vi "Perform Action.vi"(7 "Action":T1, 8 "error in (no error)":errorcluster, 11 "Item in":refnum<class "Item.lvclass">) -> (0 "error out":errorcluster, 2 "Action Performed?":bool, 3 "Item out":refnum<class "Item.lvclass">)   [LabVIEW 2020, in "Code Cleanup.lvlib" / "Item.lvclass"]
uses:
  Item.lvclass
  Item.lvclass/Item.ctl
  Code Cleanup.lvlib
  CTLs/Cleanup Action.ctl
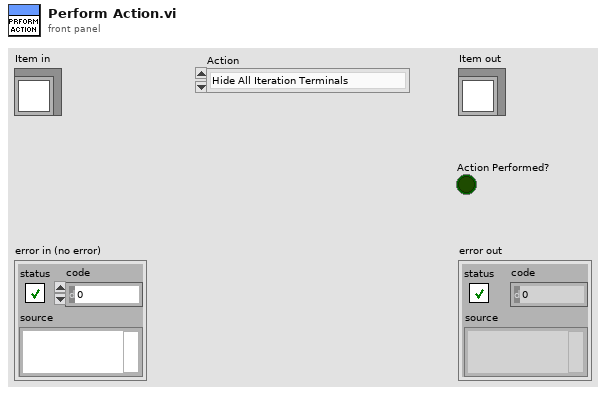
[diagram p1: front panel]
types:
  T1 = typedef "Code Cleanup.lvlib/Cleanup Action.ctl" = enum16{"Hide All Iteration Terminals", "Rename Window Title to VI Name", "Set Minimum Pane Size to (0,0)", "Set Origin to (0,0)", "Set Terminals to Required", "Fix VI Icon Properties", "Add Library Icon Layer", "Add VI Icon Layer", "Remove Icon Template", "Remove Autogrow from Structures", "Arrange Control Labels", "Format Control Labels", "Set Default FP BG Color", "Unshow Controls as Icons", "Set Modern Control Style", "Set Default Grid Sizes"}
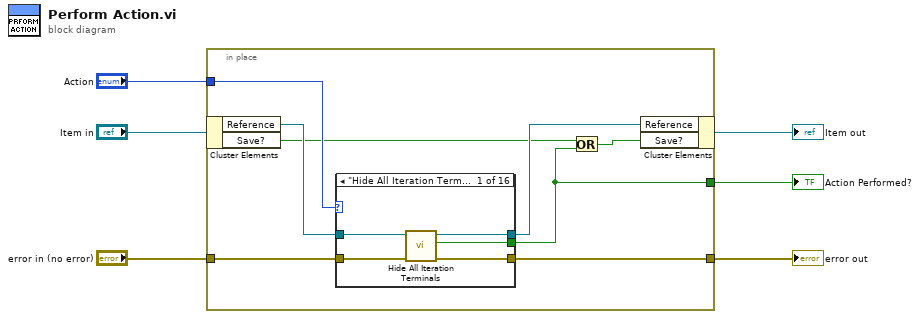
[diagram p0: block diagram]
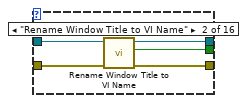
[diagram p2: hidden frame]
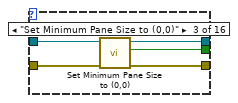
[diagram p3: hidden frame]
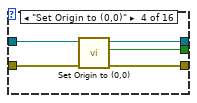
[diagram p4: hidden frame]
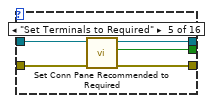
[diagram p5: hidden frame]
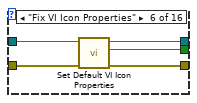
[diagram p6: hidden frame]
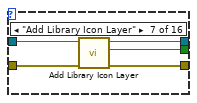
[diagram p7: hidden frame]
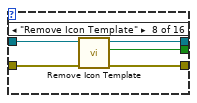
[diagram p8: hidden frame]
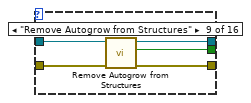
[diagram p9: hidden frame]
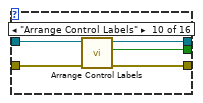
[diagram p10: hidden frame]
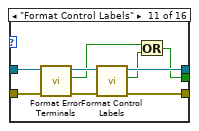
[diagram p11: hidden frame]
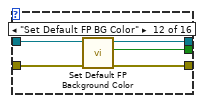
[diagram p12: hidden frame]
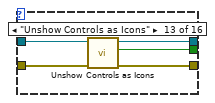
[diagram p13: hidden frame]
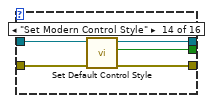
[diagram p14: hidden frame]
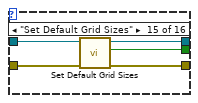
[diagram p15: hidden frame]
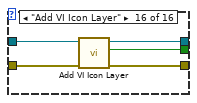
[diagram p16: hidden frame]
diagram:
  n1 = in-place {
    in-place-border: "Action" -> [w13]
    in-place-border: "error in (no error)" -> [w14]
    in-place-border: [w11] -> w2
    in-place-border: [w7] -> w1
    n2 = in-place-cluster #1("Item in") -> ("Reference"=w12:refnum<vi>, "Save?"=w9:bool)
    n3 = case shown="\"Hide All Iteration Terminals\"" w13 {
      tunnel: w14 -> [w19 w24 w29 w34 w39 w44 w49 w54 w59 w64 w72 w78 w83 w88 w93 w98]
      tunnel: w12 -> [w17 w22 w27 w32 w38 w42 w47 w52 w57 w62 w70 w76 w81 w86 w91 w96]
      tunnel: [w18 w23 w28 w33 w37 w43 w48 w53 w58 w63 w73 w77 w82 w87 w92 w97] -> w11
      tunnel: [w16 w21 w26 w31 w36 w41 w46 w51 w56 w61 w68 w75 w80 w85 w90 w95] -> w10
      tunnel: [w15 w20 w25 w30 w35 w40 w45 w50 w55 w60 w65 w74 w79 w84 w89 w94] -> w7
      frame "Hide All Iteration Terminals" {
        n4 = call "Hide All Iteration Terminals.vi"("error in (no error)"=w19, "VI Ref"=w17) -> ("error out"=w18:errorcluster, "Save?"=w15:bool, "VI Ref out"=w16:refnum<vi>)  [unwired: 7 in]
      }
      frame "Rename Window Title to VI Name" {
        n5 = call "Rename Window Title to VI Name.vi"("error in (no error)"=w24, "VI Ref"=w22) -> ("error out"=w23:errorcluster, "Save?"=w20:bool, "VI Ref out"=w21:refnum<vi>)  [unwired: 7 in]
      }
      frame "Set Minimum Pane Size to (0,0)" {
        n6 = call "Set Minimum Pane Size to (0,0).vi"("error in (no error)"=w29, "VI Ref"=w27) -> ("error out"=w28:errorcluster, "Save?"=w25:bool, "VI Ref out"=w26:refnum<vi>)  [unwired: 7 in]
      }
      frame "Set Origin to (0,0)" {
        n7 = call "Set Origin to (0,0).vi"("error in (no error)"=w34, "VI Ref"=w32) -> ("error out"=w33:errorcluster, "Save?"=w30:bool, "VI Ref out"=w31:refnum<vi>)  [unwired: 7 in]
      }
      frame "Set Terminals to Required" {
        n8 = call "Set Conn Pane Recommended to Required.vi"("error in (no error)"=w39, "VI Ref"=w38) -> ("error out"=w37:errorcluster, "Save?"=w35:bool, "VI Ref out"=w36:refnum<vi>)  [unwired: 7 in]
      }
      frame "Fix VI Icon Properties" {
        n9 = call "Set Default VI Icon Properties.vi"("error in (no error)"=w44, "VI Ref"=w42) -> ("error out"=w43:errorcluster, "Save?"=w40:bool, "VI Ref out"=w41:refnum<vi>)  [unwired: 7 in]
      }
      frame "Add Library Icon Layer" {
        n10 = call "Add Library Icon Layer.vi"("error in (no error)"=w49, "VI Ref"=w47) -> ("error out"=w48:errorcluster, "Save?"=w45:bool, "VI Ref out"=w46:refnum<vi>)  [unwired: 7 in]
      }
      frame "Remove Icon Template" {
        n11 = call "Remove Icon Template.vi"("error in (no error)"=w54, "VI Ref"=w52) -> ("error out"=w53:errorcluster, "Save?"=w50:bool, "VI Ref out"=w51:refnum<vi>)  [unwired: 7 in]
      }
      frame "Remove Autogrow from Structures" {
        n12 = call "Remove Autogrow from Structures.vi"("error in (no error)"=w59, "VI Ref"=w57) -> ("error out"=w58:errorcluster, "Save?"=w55:bool, "VI Ref out"=w56:refnum<vi>)  [unwired: 7 in]
      }
      frame "Arrange Control Labels" {
        n13 = call "Arrange Control Labels.vi"("error in (no error)"=w64, "VI Ref"=w62) -> ("error out"=w63:errorcluster, "Save?"=w60:bool, "VI Ref out"=w61:refnum<vi>)  [unwired: 7 in]
      }
      frame "Format Control Labels" {
        n14 = call "Format Error Terminals.vi"("error in (no error)"=w72, "VI Ref"=w70) -> ("error out"=w71:errorcluster, "Save?"=w66:bool, "VI Ref out"=w69:refnum<vi>)  [unwired: 7 in]
        n15 = call "Format Control Labels.vi"("error in (no error)"=w71, "VI Ref"=w69) -> ("error out"=w73:errorcluster, "Save?"=w67:bool, "VI Ref out"=w68:refnum<vi>)  [unwired: 7 in]
        n16 = Or(x=w66, y=w67) -> (x .or. y?=w65:bool)
      }
      frame "Set Default FP BG Color" {
        n17 = call "Set Default FP Background Color.vi"("error in (no error)"=w78, "VI Ref"=w76) -> ("error out"=w77:errorcluster, "Save?"=w74:bool, "VI Ref out"=w75:refnum<vi>)  [unwired: 7 in]
      }
      frame "Unshow Controls as Icons" {
        n18 = call "Unshow Controls as Icons.vi"("error in"=w83, "VI Ref"=w81) -> ("error out"=w82:errorcluster, "Save?"=w79:bool, "VI Ref out"=w80:refnum<vi>)  [unwired: 7 in]
      }
      frame "Set Modern Control Style" {
        n19 = call "Set Default Control Style.vi"("error in (no error)"=w88, "VI Ref"=w86) -> ("error out"=w87:errorcluster, "Save?"=w84:bool, "VI Ref out"=w85:refnum<vi>)  [unwired: 7 in]
      }
      frame "Set Default Grid Sizes" {
        n20 = call "Set Default Grid Sizes.vi"("error in (no error)"=w93, "VI Ref"=w91) -> ("error out"=w92:errorcluster, "Save?"=w89:bool, "VI Ref out"=w90:refnum<vi>)  [unwired: 7 in]
      }
      frame "Add VI Icon Layer" {
        n21 = call "Add VI Icon Layer.vi"("error in (no error)"=w98, "VI Ref"=w96) -> ("error out"=w97:errorcluster, "Save?"=w94:bool, "VI Ref out"=w95:refnum<vi>)  [unwired: 7 in]
      }
    }
    n22 = Or(x=w9, y=w7) -> (x .or. y?=w8:bool)
    n23 = in-place-cluster #1("Reference"=w10, "Save?"=w8) -> (→"Item out":refnum<class "Item.lvclass">)
  }
  "error out" <- w2
  "Action Performed?" <- w1
